vi "Read ini.vi"(11 "configuration file path":path caption="配置文件的路径") -> (3 "数组":string[][](array[string]))   [LabVIEW 2021]
uses:
  <vilib>/Utility/config.llb/Read Key (String).vi
  <vilib>/Utility/config.llb/NI_LVConfig.lvlib
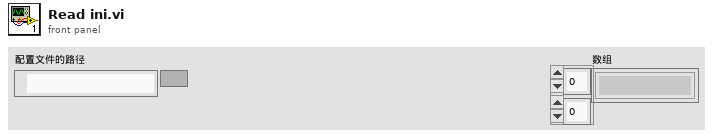
[diagram p1: front panel]
types:
  T1 = typedef "NI_LVConfig.lvlib/Config Data RefNum.ctl" = refnum<k1>
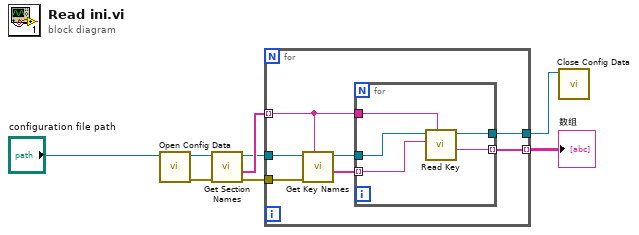
[diagram p0: block diagram]
diagram:
  n1 = call <vilib>:"Open Config Data.vi"("configuration file path"="configuration file path") -> ("error out"=w7:errorcluster, "refnum"=w6:T1)  [unwired: 8 in, 1 out]
  n2 = call <vilib>:"Get Section Names.vi"("error in (no error)"=w7, "refnum"=w6) -> ("error out"=w4:errorcluster, "section names"=w5:string[], "refnum out"=w3:T1)  [unwired: 7 in]
  n3 = for {
    tunnel: w5 -> [w11] mode=indexing
    tunnel: w4 -> [w15]
    tunnel: w3 -> [w14]
    tunnel: [w10] -> w2
    tunnel: [w9] -> w1 mode=indexing
    n4 = call <vilib>:"Get Key Names.vi"("section"=w11, "error in (no error)"=w15, "refnum"=w14) -> ("key names"=w12:string[], "refnum out"=w13:T1)  [unwired: 5 in, 2 out]
    n5 = for {
      tunnel: w13 -> [w20]
      tunnel: w12 -> [w19] mode=indexing
      tunnel: w11 -> [w18]
      tunnel: [w17] -> w10
      tunnel: [w16] -> w9 mode=indexing
      n6 = call-poly <vilib>:"Read Key.vi"("section"=w18, "key"=w19, "refnum"=w20) -> ("value"=w16:string, "refnum out"=w17:T1)  [unwired: 5 in, 2 out]
    }
  }
  "数组" <- w1
  n7 = call <vilib>:"Close Config Data.vi"("refnum"=w2) -> ()  [unwired: 9 in, 2 out]
